vi "Service Type.vi"(11 "Service in":refnum<class "Service.lvclass">) -> (2 "Type":string)   [LabVIEW 2020, in "Vecto.lvlib" / "Service.lvclass"]
uses:
  Service.lvclass
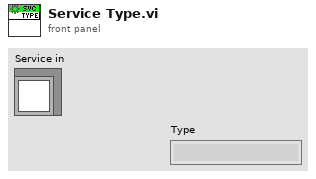
[diagram p1: front panel]
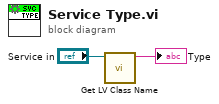
[diagram p0: block diagram]
diagram:
  n1 = call <vilib>:"Get LV Class Name.vi"("object"="Service in") -> ("class name"=→"Type":string)  [unwired: 9 in, 1 out]
